vi "LaunchBall.vi"(8 "error in (no error)":errorcluster) -> (0 "error out":errorcluster)   [LabVIEW 2013]
uses:
  Global.vi
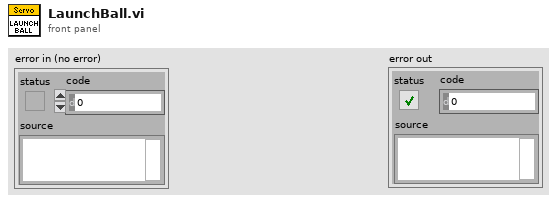
[diagram p1: front panel]
types:
  T1 = typedef "WPI_ServoDeviceRef.ctl" = cluster{"DeviceStatus":errorcluster, "Digital Module":T2, "PWM Channel":T3, "DeadBand":T4}
  T2 = typedef "FPGA_TypedefDigitalModule.ctl" = enum16{"Digital Module 1", "Digital Module 2"}
  T3 = typedef "FPGA_DIOPWMChannel.ctl" = enum8{"PWM 1", "PWM 2", "PWM 3", "PWM 4", "PWM 5", "PWM 6", "PWM 7", "PWM 8", "PWM 9", "PWM 10", "Invalid"}
  T4 = typedef "WPI_PWMDeadband.ctl" = cluster{"Name":string, "maxPositivePwm":i32, "minPositivePwm":i32, "centerPwm":i32, "maxNegativePwm":i32, "minNegativePwm":i32, "angularRange":u16}
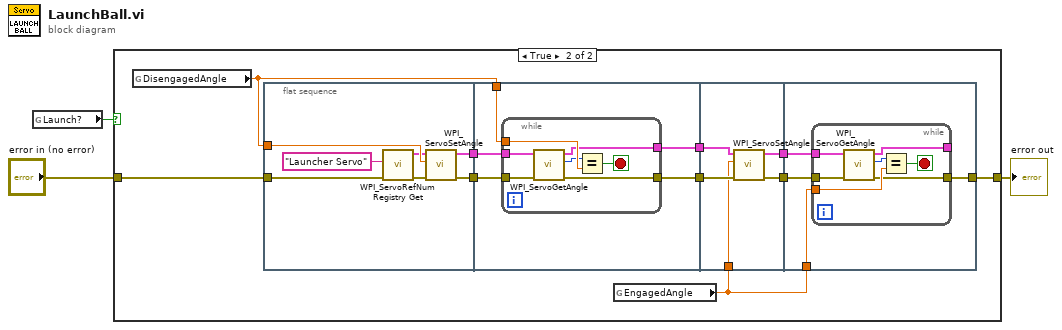
[diagram p0: block diagram]
diagram:
  n1 = global read "Global.vi" "Launch?"() -> (w3:bool)
  n2 = case shown="True" w3 {
    tunnel: "error in (no error)" -> [w4 w14]
    tunnel: [w4 w8] -> w1
    frame False {
    }
    frame True {
      n3 = global read "Global.vi" "DisengagedAngle"() -> (w11:dbl)
      n4 = flat-sequence {
        tunnel: w11 -> [w21]
        tunnel: w14 -> [w20]
        tunnel: [w17] -> w13
        tunnel: [w15] -> w12
        tunnel: w13 -> [w26]
        tunnel: w12 -> [w25]
        tunnel: w11 -> [w24]
        tunnel: [w23] -> w10
        tunnel: [w22] -> w9
        tunnel: w10 -> [w38]
        tunnel: w9 -> [w37]
        tunnel: w6 -> [w36]
        tunnel: [w35] -> w7
        tunnel: [w34] -> w5
        tunnel: [w41] -> w8
        tunnel: w7 -> [w42]
        tunnel: w6 -> [w40]
        tunnel: w5 -> [w39]
        frame #0 {
          n5 = call <vilib>:"WPI_ServoRefNum Registry Get.vi"("error in (no error)"=w20, "refnum name"="Launcher Servo") -> ("error out"=w19:errorcluster, "ServoDeviceRef"=w16:T1)  [unwired: 8 in]
          n6 = call <vilib>:"WPI_ServoSetAngle.vi"("error in (no error)"=w19, "Angle"=w21, "ServoDeviceRef"=w16) -> ("error out"=w17:errorcluster, "ServoDeviceRef"=w15:T1)  [unwired: 7 in]
        }
        frame #1 {
          n7 = while {
            tunnel: w26 -> [w33]
            tunnel: w25 -> [w32]
            tunnel: w24 -> [w31]
            tunnel: [w28] -> w23
            tunnel: [w27] -> w22
            stop <- w29 stop-if-true
            n8 = call <vilib>:"WPI_ServoGetAngle.vi"("ServoDeviceRef"=w32, "error in (no error)"=w33) -> ("ServoDeviceRef"=w28:T1, "Angle"=w30:u16, "error out"=w27:errorcluster)  [unwired: 6 in]
            n9 = Equal?(x=w30, y=w31) -> (x = y?=w29:bool)
          }
        }
        frame #2 {
          n10 = call <vilib>:"WPI_ServoSetAngle.vi"("error in (no error)"=w37, "Angle"=w36, "ServoDeviceRef"=w38) -> ("error out"=w35:errorcluster, "ServoDeviceRef"=w34:T1)  [unwired: 7 in]
        }
        frame #3 {
          n11 = while {
            tunnel: w42 -> [w49]
            tunnel: w39 -> [w48]
            tunnel: w40 -> [w47]
            tunnel: [w44] -> _
            tunnel: [w43] -> w41
            stop <- w45 stop-if-true
            n12 = call <vilib>:"WPI_ServoGetAngle.vi"("ServoDeviceRef"=w48, "error in (no error)"=w49) -> ("ServoDeviceRef"=w44:T1, "Angle"=w46:u16, "error out"=w43:errorcluster)  [unwired: 6 in]
            n13 = Equal?(x=w46, y=w47) -> (x = y?=w45:bool)
          }
        }
      }
      n14 = global read "Global.vi" "EngagedAngle"() -> (w6:dbl)
    }
  }
  "error out" <- w1
